vi "Draw.vi"() -> ()   [LabVIEW 2014]
doc: "Use this template to build a VI to use as a subVI."
uses:
  <vilib>/vision/NI_Vision_Development_Module.lvlib
panel:
  out "Img":T1(plugin-control)
  # ":: MVi Framework V1.0 ::\nAuthor:Gaoke Yang\nEmail: gaoke.yang@yahoo.com\nWeb: www.mvicontrol.com\nCopyright (C) 2015, MVI Technologies All Rights Reserved"
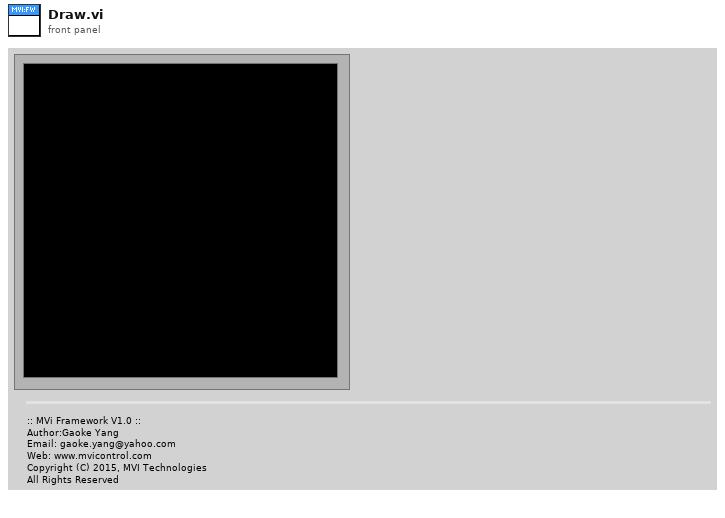
[diagram p1: front panel]
types:
  T1 = typedef "IMAQ Image.ctl" = refnum<image>
  T2 = cluster{"Desired Font (Application)":enum16{"User-specified Font", "Application Font", "System Font", "Dialog Font"}, "[User-specified Font]":cluster{"Font Name":string, "Size":i16, "Strikeout?":bool, "Italic?":bool, "Underline?":bool, "Outline?":bool, "Shadow?":bool, "Bold?":bool, "Rotation Angle":dbl}, "Horizontal Alignment":i16, "Vertical Alignment":i16}
  T3 = typedef "Image Type" = u32
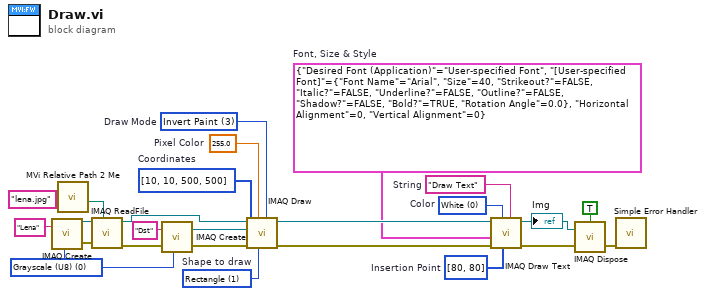
[diagram p0: block diagram]
diagram:
  w1 = i32[] [80, 80]  # Insertion Point
  w2 = T2 {"Desired Font (Application)"=enum."User-specified Font", "[User-specified Font]"={"Font Name"="Arial", "Size"=40, "Strikeout?"=FALSE, "Italic?"=FALSE, "Underline?"=FALSE, "Outline?"=FALSE, "Shadow?"=FALSE, "Bold?"=TRUE, "Rotation Angle"=0.0}, "Horizontal Alignment"=0, "Vertical Alignment"=0}  # Font, Size & Style
  w3 = 0 items=["White", "Black", "Inverted", "Black on White", "White on Black"]  # Color
  w4 = "Draw Text"  # String
  w7 = u16 3 items=["Frame", "Paint", "Invert Frame", "Invert Paint"]  # Draw Mode
  w8 = sgl 255.0  # Pixel Color
  w9 = i32[] [10, 10, 500, 500]  # Coordinates
  w10 = u16 1 items=["Line", "Rectangle", "Oval"]  # Shape to draw
  w14 = T3 0 items=["Grayscale (U8)", "Grayscale (I16)", "Grayscale (SGL)", "Complex (CSG)", "RGB (U32)", "HSL (U32)", "RGB (U64)", "Grayscale (U16)"] ("Image Type")
  n1 = call "IMAQ Create"("Image Name"="Lena" ("name or relative path"), "Image Type"=w14) -> ("New Image"=w25:T1, "error out"=w24:errorcluster)  [unwired: 2 in, 1 out]
  n2 = call "MVi Relative Path 2 Me.vi"("Relative Path"="lena.jpg" ("name or relative path")) -> ("Appended Dir"=w19:path)  [unwired: 5 in, 1 out]
  n3 = call "IMAQ ReadFile"("File Path"=w19, "error in (no error)"=w24, "Image"=w25) -> ("error out"=w12:errorcluster, "Image Out"=w16:T1)  [unwired: 4 in, 3 out]
  n4 = call "IMAQ Create"("Image Name"="Dst" ("name or relative path"), "Image Type"=w14, "error in (no error)"=w12) -> ("New Image"=w13:T1, "error out"=w11:errorcluster)  [unwired: 1 in, 1 out]
  n5 = call "IMAQ Draw"("Draw Mode"=w7, "Shape to draw"=w10, "Pixel Color"=w8, "error in (no error)"=w11, "Coordinates"=w9, "Image Dst"=w13, "Image Src"=w16) -> ("error out"=w18:errorcluster, "Image Dst Out"=w6:T1)  [unwired: 3 in]
  n6 = call "IMAQ Draw Text"("String"=w4, "Insertion Point"=w1, "Color"=w3, "error in (no error)"=w18, "Font, Size & Style"=w2, "Image Src"=w6) -> ("error out"=w17:errorcluster, "Image Dst Out"=w5:T1)  [unwired: 2 in, 2 out]
  "Img" <- w5
  n7 = call "IMAQ Dispose"("All Images? (No)"=TRUE, "Image"=w5, "error in (no error)"=w17) -> ("error out"=w20:errorcluster)  [unwired: 3 out]
  n8 = call <vilib>:"Simple Error Handler.vi"("error in (no error)"=w20) -> ()  [unwired: 1 in, 8 out]
